vi "Launch Base Queue.vi"(9 "Queue jettl":refnum<class "Queue jettl.lvclass">, 10 "Alias":string) -> (0 "error out":errorcluster)   [LabVIEW 2021, in "jettl.lvlib" / "Base Queue jettl.lvlib"]
uses:
  Base Queue jettl.lvlib
  Queue jettl/Queue jettl.lvclass
  Base Queue jettl/Base Queue jettl.lvclass
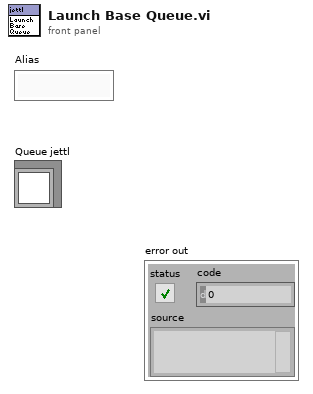
[diagram p1: front panel]
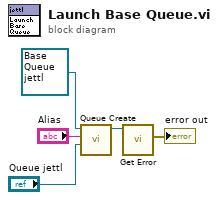
[diagram p0: block diagram]
diagram:
  n1 = call-dynamic "Queue Create.vi"("Queue jettl"="Queue jettl", "Alias"="Alias", "Base Queue jettl in"=refnum<class "Base Queue jettl.lvclass"> refnum ("jettl Queue Actor.lvlib:jettl Queue Actor.lvclass")) -> ("Base Queue jettl out"=w4:refnum<class "Base Queue jettl.lvclass">)  [unwired: 8 in]
  n2 = call-dynamic "Get Error.vi"("Base Queue jettl in"=w4) -> ("Error"=→"error out":errorcluster)  [unwired: 10 in]
